vi "config_step_motor.vi"(11 "step_motor_data":T1={"SerialPort"="", "MinTime"=0.0, "baud rate"=9600, "data bits"=8, "parity"=enum."None", "stop bits"=10, "flow control"=0, "Steps"=0, "Active"=FALSE} {"flow control" items=["None", "XON/XOFF", "RTS/CTS", "XON/XOFF & RTS/CTS", "DTR/DSR", "XON/XOFF & DTR/DSR"]; "stop bits" items=["1.0"=10, "1.5"=15, "2.0"=20]; "data bits" min=5 max=8 step=1}) -> (3 "step_motor_data out":T1={"SerialPort"="", "MinTime"=0.0, "baud rate"=9600, "data bits"=8, "parity"=enum."None", "stop bits"=10, "flow control"=0, "Steps"=0, "Active"=FALSE} {"flow control" items=["None", "XON/XOFF", "RTS/CTS", "XON/XOFF & RTS/CTS", "DTR/DSR", "XON/XOFF & DTR/DSR"]; "stop bits" items=["1.0"=10, "1.5"=15, "2.0"=20]; "data bits" min=5 max=8 step=1})   [LabVIEW 2016]
uses:
  step_motor_data.ctl
panel:
  in  "MinTime":dbl=0.1 caption="Tempo mínimo entre passos [s]"
  in  "Porta serial":refnum<visa-resource-name>="COM5"
  in  "OK":bool
  in  "flow control":u16(ring) items=["None"=0, "XON/XOFF"=1, "RTS/CTS"=2, "DTR/DSR"=4]
  in  "stop bits":u16(ring)=10 items=["1.0"=10, "1.5"=15, "2.0"=20]
  in  "parity":enum16{"None", "Odd", "Even", "Mark", "Space"}(ring)
  in  "data bits":u16=8 min=5 max=8 step=1
  in  "baud rate":u32(ring)=57600 items=["75"=75, "110"=110, "134"=134, "150"=150, "300"=300, "600"=600, "1200"=1200, "1800"=1800, "2400"=2400, "4800"=4800, "7200"=7200, "9600"=9600, "14400"=14400, "19200"=19200, "28800"=28800, "38400"=38400, "56000"=56000, "57600"=57600, "115200"=115200, "128000"=128000, "230400"=230400]
  # "Configuração do motor de passo"
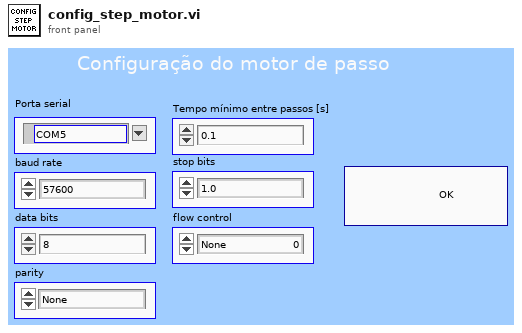
[diagram p1: front panel]
types:
  T1 = typedef "step_motor_data.ctl" = cluster{"SerialPort":refnum<visa-resource-name>, "MinTime":dbl, "baud rate":u32, "data bits":u16, "parity":enum16{"None", "Odd", "Even", "Mark", "Space"}, "stop bits":u16, "flow control":u16, "Steps":i32, "Active":bool}
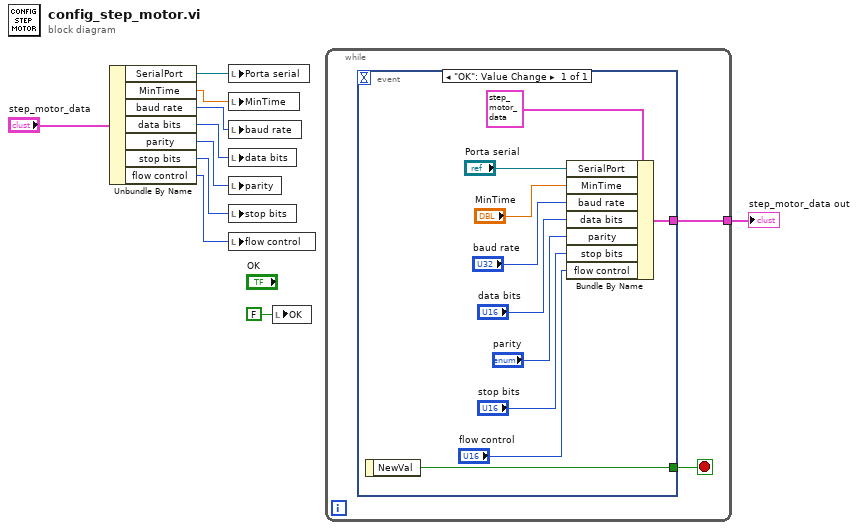
[diagram p0: block diagram]
diagram:
  n1 = Unbundle By Name("step_motor_data") -> ("SerialPort"=w7:refnum<visa-resource-name>, "MinTime"=w6:dbl, "baud rate"=w5:u32, "data bits"=w4:u16, "parity"=w3:enum16{"None", "Odd", "Even", "Mark", "Space"}, "stop bits"=w2:u16, "flow control"=w1:u16)
  n2 = local write "Porta serial"(w7) -> ()
  n3 = local write "MinTime"(w6) -> ()
  n4 = local write "baud rate"(w5) -> ()
  n5 = local write "data bits"(w4) -> ()
  n6 = local write "parity"(w3) -> ()
  n7 = local write "stop bits"(w2) -> ()
  n8 = local write "flow control"(w1) -> ()
  n9 = local write "OK"(FALSE ("OK")) -> ()
  n10 = while {
    tunnel: [w11] -> w9
    stop <- w12 stop-if-true
    n11 = event shown="[0] \"OK\": Value Change" {
      selector: _ -> [_]
      dyn-events: _ -> [_]
      timeout: _ -> [_]
      tunnel: [w22] -> w12
      tunnel: [w13] -> w11
      event "OK": Value Change {
        n12 = event-data() -> ("NewVal"=w22:bool)  [unwired: 1 in]
        n13 = Bundle By Name(cluster=T1 {"SerialPort"="", "MinTime"=0.0, "baud rate"=57600, "data bits"=8, "parity"=enum."None", "stop bits"=10, "flow control"=0, "Steps"=0, "Active"=FALSE} ("step_motor_data"), "SerialPort"="Porta serial", "MinTime"="MinTime", "baud rate"="baud rate", "data bits"="data bits", "parity"="parity", "stop bits"="stop bits", "flow control"="flow control") -> (w13:T1)
      }
    }
  }
  "step_motor_data out" <- w9
